vi "Create Directory if Necessary.vi"(8 "error in":errorcluster, 11 "File Path":path) -> (0 "error out":errorcluster)   [LabVIEW 2014, in "RunVIAnalyzer.lvclass"]
uses:
  RunVIAnalyzer.lvclass
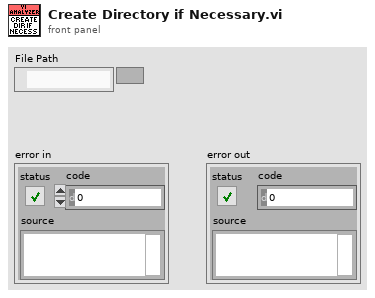
[diagram p1: front panel]
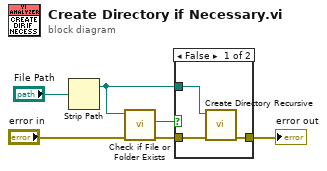
[diagram p0: block diagram]
diagram:
  n1 = Strip Path(path="File Path") -> (stripped path=w1:path)  [unwired: 1 out]
  n2 = call <vilib>:"Check if File or Folder Exists.vi"("error in (no error)"="error in", "path"=w1) -> ("error out"=w4:errorcluster, "file or folder exists?"=w2:bool)  [unwired: 7 in, 1 out]
  n3 = case shown="False" w2 {
    tunnel: [w9 w10] -> w6
    tunnel: w4 -> [w8 w10]
    tunnel: w1 -> [w7 _]
    frame False {
      n4 = call <vilib>:"Create Directory Recursive.vi"("error in (no error)"=w8, "directory"=w7) -> ("error out"=w9:errorcluster)  [unwired: 3 in, 2 out]
    }
    frame True {
    }
  }
  "error out" <- w6
